vi "Init Nested Actors.vi"(8 "error in (no error)":errorcluster, 11 "Coffee Shop in":refnum<class "Coffee Shop.lvclass">) -> (0 "error out":errorcluster, 3 "Coffee Shop out":refnum<class "Coffee Shop.lvclass">)   [LabVIEW 2023, in "Coffee Shop.lvlib" / "Coffee Shop.lvclass"]
doc: "Launch the nested actors that the system requires at start-up."
uses:
  Coffee Shop.lvclass
  c:/dev/_r/4/eng/lv-core/lvpostprocessingd/lv_mc_x86_64/dist_i386/vi.lib/ActorFramework/Actor/Actor.lvclass
  Work Dispatcher/Work Dispatcher.lvclass
  <vilib>/ActorFramework/Actor/Actor.lvclass/Actor.ctl
  <vilib>/ActorFramework/Message Enqueuer/Message Enqueuer.lvclass/Message Enqueuer.ctl
  Coffee Shop.lvclass/Coffee Shop.ctl
  <vilib>/ActorFramework/Message Enqueuer/Init from Existing Queue.vi
  <vilib>/ActorFramework/Message Enqueuer/Enqueue.vi
  Coffee Shop Messages/Add Barista Msg/Add Barista Msg.lvclass
  c:/dev/_r/4/eng/lv-core/lvpostprocessingd/lv_mc_x86_64/dist_i386/vi.lib/ActorFramework/Message/Message.lvclass
  Coffee Shop Messages/Add Cashier Msg/Add Cashier Msg.lvclass
  <vilib>/ActorFramework/Message Priority Queue/Priority Enqueue.vi
  <vilib>/ActorFramework/Message Enqueuer/Message Enqueuer.lvclass
  <vilib>/ActorFramework/Actor/Actor.lvclass
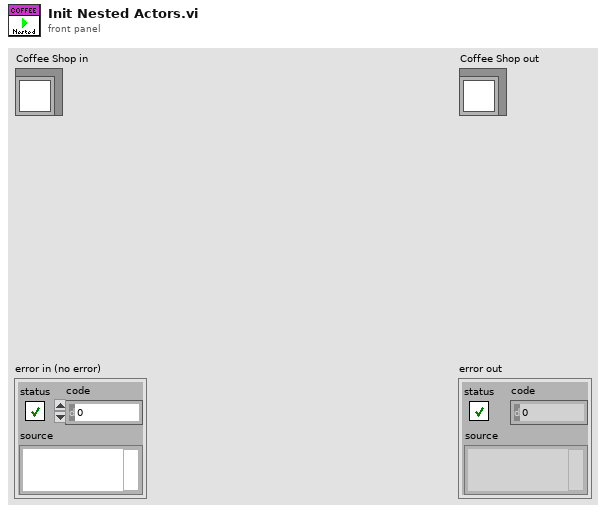
[diagram p1: front panel]
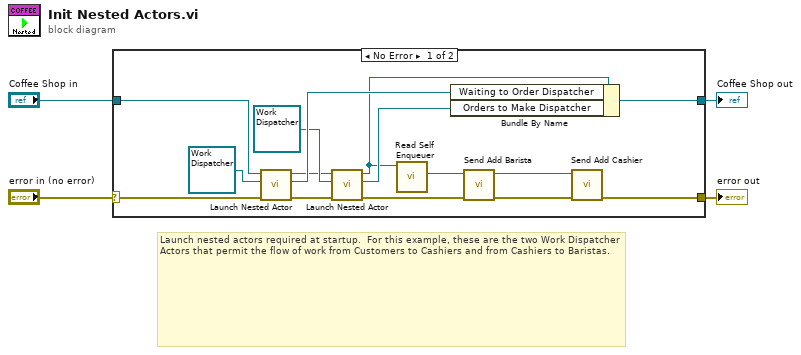
[diagram p0: block diagram]
diagram:
  # "Launch nested actors required at startup.  For this example, these are the two Work Dispatcher Actors that permit the flow of work from Customers to Cashiers and from Cashiers to Baristas."
  n1 = case shown="No Error" "error in (no error)" {
    selector: "error in (no error)" -> [w19 w21]
    tunnel: [w18 w21] -> w3
    tunnel: [w17 w20] -> w1
    tunnel: "Coffee Shop in" -> [w10 w20]
    frame No Error {
      n2 = call <vilib>:"Launch Nested Actor.vi"("error in (no error)"=w19, "Nested Actor"=refnum<class "Work Dispatcher.lvclass"> refnum ("Work Dispatcher.lvclass"), "Caller Actor in"=w10) -> ("error out"=w16:errorcluster, "Nested Actor's Enqueuer"=w14:refnum<class "Message Enqueuer.lvclass">, "Caller Actor out"=w8:refnum<class "Coffee Shop.lvclass">)  [unwired: 6 in]
      n3 = call <vilib>:"Launch Nested Actor.vi"("error in (no error)"=w16, "Nested Actor"=refnum<class "Work Dispatcher.lvclass"> refnum ("Work Dispatcher.lvclass"), "Caller Actor in"=w8) -> ("error out"=w15:errorcluster, "Nested Actor's Enqueuer"=w13:refnum<class "Message Enqueuer.lvclass">, "Caller Actor out"=w7:refnum<class "Coffee Shop.lvclass">)  [unwired: 6 in]
      n4 = call <vilib>:"Read Self Enqueuer.vi"("Actor"=w7) -> ("Self Enqueuer"=w12:refnum<class "Message Enqueuer.lvclass">)  [unwired: 10 in]
      n5 = Bundle By Name(cluster=w7, "Waiting to Order Dispatcher"=w14, "Orders to Make Dispatcher"=w13) -> (w17:refnum<class "Coffee Shop.lvclass">)
      n6 = call "Send Add Barista.vi"("error in (no error)"=w15, "Message Enqueuer"=w12) -> ("error out"=w5:errorcluster, "Message Enqueuer out"=w6:refnum<class "Message Enqueuer.lvclass">)  [unwired: 8 in]
      n7 = call "Send Add Cashier.vi"("error in (no error)"=w5, "Message Enqueuer"=w6) -> ("error out"=w18:errorcluster)  [unwired: 8 in, 1 out]
    }
    frame Error {
    }
  }
  "error out" <- w3
  "Coffee Shop out" <- w1
